vi "Transfer Group Info to Command.vi"(8 "error in (no error)":errorcluster, 9 "Transfer Group iteration":u64, 10 "Transfer Group id":i32, 11 "Transceiver Thread in":refnum<class "Transceiver Thread.lvclass">) -> (0 "error out":errorcluster, 2 "command parameters":T1, 3 "Transceiver Thread out":refnum<class "Transceiver Thread.lvclass">)   [LabVIEW 2017, in "Data Sharing Framework Engine.lvlib" / "Transceiver Thread.lvclass"]
uses:
  Transceiver Thread.lvclass
  Interfaces/Transceiver Interface/Command Parameters.ctl
  Interfaces/Transceiver Interface/Transceiver Interface.lvclass
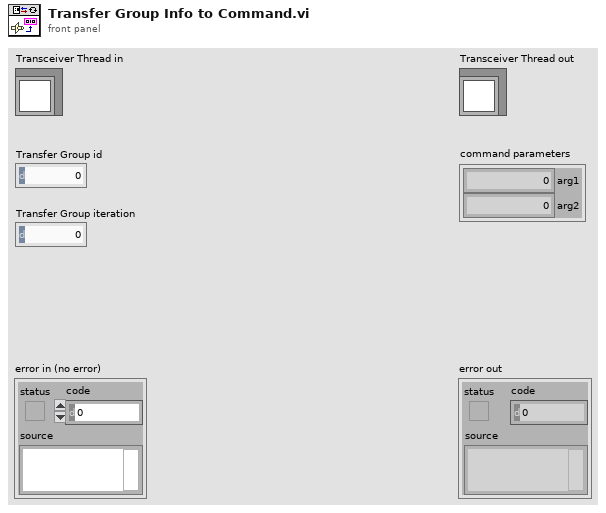
[diagram p1: front panel]
types:
  T1 = typedef "Data Sharing Framework Engine.lvlib/Transceiver Interface.lvclass/Command Parameters.ctl" = cluster{"arg1":u64, "arg2":u64}
  T2 = cluster{"Transfer Group ID":i32, "unused":i32, "Transfer Group iteration":u64}
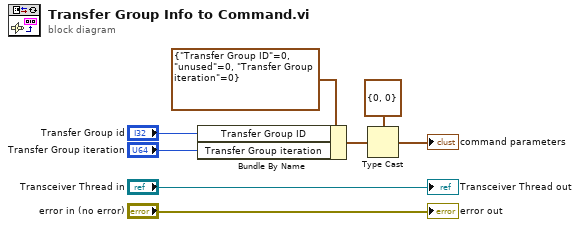
[diagram p0: block diagram]
diagram:
  n1 = Bundle By Name(cluster=T2 {"Transfer Group ID"=0, "unused"=0, "Transfer Group iteration"=0} ("Cluster"), "Transfer Group ID"="Transfer Group id", "Transfer Group iteration"="Transfer Group iteration") -> (w3:T2)
  n2 = Type Cast(type=T1 {"arg1"=0, "arg2"=0} ("command parameters"), x=w3) -> (*(type *) &x=→"command parameters":T1)
  "error out" <- "error in (no error)"
  "Transceiver Thread out" <- "Transceiver Thread in"
